vi "StopScanMessage.vi"() -> (3 "StopScanMessage":string)   [LabVIEW 2019]
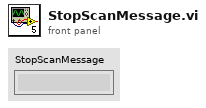
[diagram p1: front panel]
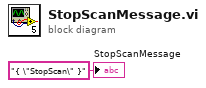
[diagram p0: block diagram]
diagram:
  "StopScanMessage" <- "{ \"StopScan\" }" ("StopScanMessage")
